vi "Configure Trigger Out.vi"(8 "error in (no error)":errorcluster, 9 "Output Trigger Enable (T: On)":bool=TRUE, 10 "Output Trigger Slope (F: Negative)":bool, 11 "VISA resource name":refnum<visa-resource-name>) -> (0 "error out":errorcluster, 3 "VISA resource name out":refnum<visa-resource-name>)   [LabVIEW 2017, in "Keithley 3390.lvlib"]
doc: "Configures the function generator's output trigger. Trigger out is used with burst mode to syncronize with the output of the burst."
uses:
  Keithley 3390.lvlib
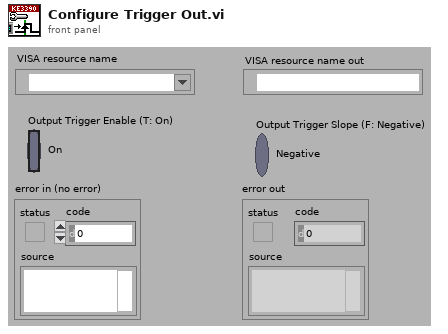
[diagram p1: front panel]
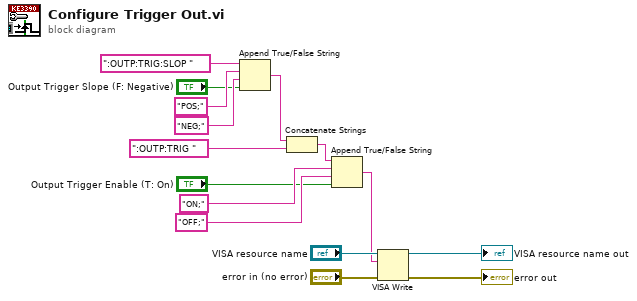
[diagram p0: block diagram]
diagram:
  n1 = Append True/False String(1:"Output Trigger Slope (F: Negative)", 2:"NEG;" ("false string"), 3:"POS;" ("true string"), 4:":OUTP:TRIG:SLOP " ("command")) -> (0:w11:string)
  n2 = Concatenate Strings(w11, ":OUTP:TRIG " ("command")) -> (w5:string)
  n3 = Append True/False String(1:"Output Trigger Enable (T: On)", 2:"OFF;" ("false string"), 3:"ON;" ("true string"), 4:w5) -> (0:w3:string)
  n4 = VISA Write(VISA resource name="VISA resource name", write buffer=w3, error in (no error)="error in (no error)") -> (VISA resource name out=→"VISA resource name out":refnum<visa-resource-name>, error out=→"error out":errorcluster)  [unwired: 1 out]
